vi "Maintain RPM.vi"(1 "Desired RPM":dbl, 2 "RPM":dbl) -> (0 "Set Motor":dbl)   [LabVIEW 2015]
panel:
  out "SeeSaw":dbl
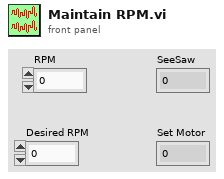
[diagram p1: front panel]
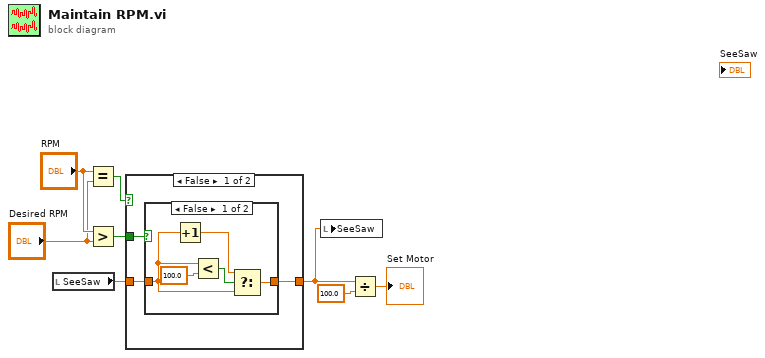
[diagram p0: block diagram]
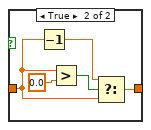
[diagram p2: hidden frame]
diagram:
  n1 = local read "SeeSaw"() -> (w3:dbl)
  n2 = Equal?(x="RPM", y="Desired RPM") -> (x = y?=w8:bool)
  n3 = Greater?(x="RPM", y="Desired RPM") -> (0:w5:bool)
  n4 = case shown="False" w8 {
    tunnel: w3 -> [w11 w22]
    tunnel: w5 -> [w9 _]
    tunnel: [w10 w22] -> w1
    frame False {
      n5 = case shown="False" w9 {
        tunnel: [w13 w18] -> w10
        tunnel: w11 -> [w12 w17]
        frame False {
          n6 = Increment(x=w12) -> (x+1=w14:dbl)
          n7 = Less?(x=w12, y=100.0) -> (x < y?=w15:bool)
          n8 = Select(t=w14, s=w15, f=w12) -> (s? t:f=w13:dbl)
        }
        frame True {
          n9 = Decrement(x=w17) -> (x-1=w19:dbl)
          n10 = Greater?(x=w17, y=0.0) -> (0:w20:bool)
          n11 = Select(t=w19, s=w20, f=w17) -> (s? t:f=w18:dbl)
        }
      }
    }
    frame True {
    }
  }
  n12 = local write "SeeSaw"(w1) -> ()
  n13 = Divide(x=w1, y=100.0) -> (x/y=→"Set Motor":dbl)
